vi "VI Ref Global.vi"() -> ()   [LabVIEW 2016]
panel:
  out "TopLevelRef":refnum<vi>
  out "PanelRef":refnum<vi>
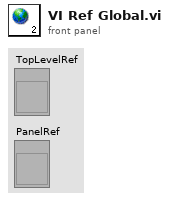
[diagram p1: front panel]
diagram:
